vi "te_getTime.vi"(1 "Current Time":timestamp) -> (11 "Seconds from Midnight":u32, 13 "Fractional Seconds":dbl, 14 "Year":u32, 15 "Month":u32, 16 "Day":u32, 17 "Hour":u32, 18 "Minutes":u32, 19 "Seconds":u32)   [LabVIEW 2018]
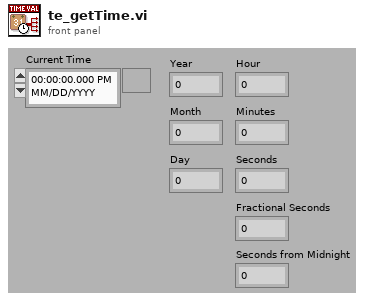
[diagram p1: front panel]
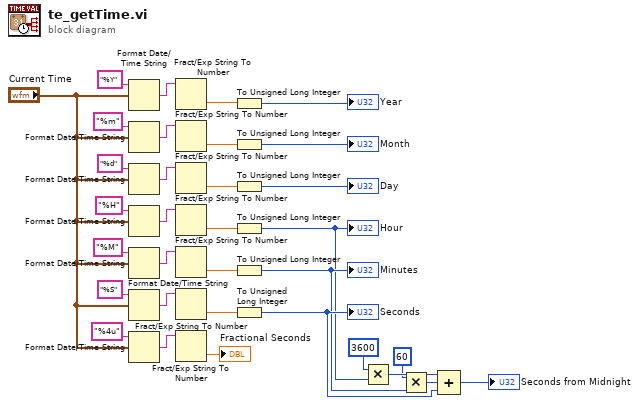
[diagram p0: block diagram]
diagram:
  n1 = Format Date/Time String(time format string (%c)="%Y", seconds (now)="Current Time") -> (date/time string=w32:string)  [unwired: 1 in]
  n2 = Format Date/Time String(time format string (%c)="%m", seconds (now)="Current Time") -> (date/time string=w30:string)  [unwired: 1 in]
  n3 = Format Date/Time String(time format string (%c)="%d", seconds (now)="Current Time") -> (date/time string=w27:string)  [unwired: 1 in]
  n4 = Format Date/Time String(time format string (%c)="%H", seconds (now)="Current Time") -> (date/time string=w29:string)  [unwired: 1 in]
  n5 = Format Date/Time String(time format string (%c)="%M", seconds (now)="Current Time") -> (date/time string=w20:string)  [unwired: 1 in]
  n6 = Format Date/Time String(time format string (%c)="%S", seconds (now)="Current Time") -> (date/time string=w22:string)  [unwired: 1 in]
  n7 = Format Date/Time String(time format string (%c)="%4u", seconds (now)="Current Time") -> (date/time string=w24:string)  [unwired: 1 in]
  n8 = Fract/Exp String To Number(string=w32) -> (number=w14:dbl)  [unwired: 3 in, 1 out]
  n9 = Fract/Exp String To Number(string=w30) -> (number=w13:dbl)  [unwired: 3 in, 1 out]
  n10 = Fract/Exp String To Number(string=w27) -> (number=w12:dbl)  [unwired: 3 in, 1 out]
  n11 = Fract/Exp String To Number(string=w29) -> (number=w11:dbl)  [unwired: 3 in, 1 out]
  n12 = Fract/Exp String To Number(string=w20) -> (number=w10:dbl)  [unwired: 3 in, 1 out]
  n13 = Fract/Exp String To Number(string=w22) -> (number=w9:dbl)  [unwired: 3 in, 1 out]
  n14 = Fract/Exp String To Number(string=w24) -> (number=→"Fractional Seconds":dbl)  [unwired: 3 in, 1 out]
  n15 = To Unsigned Long Integer(number=w14) -> (unsigned 32bit integer=→"Year":u32)
  n16 = To Unsigned Long Integer(number=w13) -> (unsigned 32bit integer=→"Month":u32)
  n17 = To Unsigned Long Integer(number=w12) -> (unsigned 32bit integer=→"Day":u32)
  n18 = To Unsigned Long Integer(number=w11) -> (unsigned 32bit integer=w2:u32)
  "Hour" <- w2
  n19 = To Unsigned Long Integer(number=w10) -> (unsigned 32bit integer=w3:u32)
  "Minutes" <- w3
  n20 = To Unsigned Long Integer(number=w9) -> (unsigned 32bit integer=w4:u32)
  "Seconds" <- w4
  n21 = Multiply(x=u32 3600 ("y"), y=w2) -> (x*y=w8:u32)
  n22 = Multiply(x=u32 60 ("y"), y=w3) -> (x*y=w7:u32)
  n23 = Compound Arithmetic op=ADD(w8, w7, w4) -> (→"Seconds from Midnight":u32)
